vi "Gel Tugging Displacement Mode v.16.00.vi"() -> ()   [LabVIEW 2015]
doc: "This example demonstrates how to continuously acquire voltage measurements from a DAQmx device using hardware timed, single point reads using a timed loop structure. The timed loop is controlled by the sample clock of the DAQ device. The device will read data on each tick of the sample clock. If an additional sample clock tick occurs before the current data point is read from the device or if the timed loop does not receive any sample clock ticks, a dialog will indicate that this has happened. \n\nHardware Timed Single Point acquisition works best when using a deterministic operating system (such as LabVIEW Real-Time). Because of the less deterministic nature of general purpose operating systems (such as Microsoft Windows), the software loop will not always take the exact same amount of time to execute, and this may lead to the occasional missed sample clock. \n\nFor instructions on how to connect your signals to the DAQ device, refer to your device documentation."
uses:
  <vilib>/Platform/TimedLoop/XDataNode/timing_clust.ctl
  <vilib>/Platform/TimedLoop/XDataNode/nitl_modes.ctl
  <vilib>/Platform/TimedLoop/XDataNode/wakeup.ctl
  <vilib>/DAQmx/read.llb/DAQmx Read (Analog 1D DBL NChan 1Samp).vi
  <vilib>/DAQmx/write.llb/DAQmx Write (Analog DBL 1Chan 1Samp).vi
  <vilib>/DAQmx/read.llb/DAQmx Read (Analog 2D DBL NChan NSamp).vi
  <vilib>/Analysis/baseanly.llb/Mean (DBL).vi
  <vilib>/DAQmx/create/channels.llb/DAQmx Create Channel (AI-Voltage-Basic).vi
  <vilib>/DAQmx/create/channels.llb/DAQmx Create Channel (AO-Voltage-Basic).vi
  <vilib>/DAQmx/configure/timing.llb/DAQmx Timing (Sample Clock).vi
  <vilib>/DAQmx/create/timing.llb/DAQmx Create Timing Source (Control Loop From Task).vi
  <vilib>/DAQmx/miscellaneous.llb/DAQmx Fill In Error Info.vi
  <vilib>/addons/control/pid/pid.llb/PID (DBL).vi
  <vilib>/platform/TimedLoop/XDataNode/XDataNode.xnode
  <vilib>/Analysis/NI_AALBase.lvlib
  <vilib>/addons/control/pid/NI_PID_pid.lvlib
  <vilib>/Platform/TimedLoop/XDataNode/XDNodeRunTimeDep.lvlib
  <vilib>/ptbypt/NI_PtbyPt.lvlib
panel:
  out "Calibrating Sensor":bool
  out "Waveform Graph":dbl[](graph)
  in  "2. Force Clamp?":bool
  in  "Measure Flux Sensor Zero?":bool=TRUE
  in  "4. Aggressiveness:":i32(listbox)
  out "of":i32
  in  "3. PID Parameters:":i32(listbox)
  out "Measured Magnetic Sensor 1 Zero, Mean (V)":dbl format="%_7g"
  out "Round:":i32
  out "Ready?":bool
  out "Sensor Sensitivity \n(V/Gs)":dbl
  in  "1. Sensor:":i32(listbox)
  out "Ready?":bool
  in  "2. Needle:":i32(listbox)
  in  "Proceed with Selection":bool
  out "Real-Time Flux Control Currently Running?":bool
  out "DeGaussing?":bool
  in  "Start DeGaussing":bool
  in  "Start Null Flux Adjustment":bool
  in  "1. Number of rounds":i32=2
  in  "3. Keep Null Flux Running \n       Until Next Step?":bool=TRUE
  in  "4. Stop Program":bool
  # "For Gel Tugging Experiments v16.00 (Force Clamp/Controlled Displacement Mode)"
  # "WARNING: This program crashes the first 2 or 3 times it runs after the target has been shut down. \nWARNING: Do NOT run the power supply unattended with the needle attached. Always look at the amount of current periodically."
  # "Step 0-1: Place the needle at Z ~ 5000 micron in the field of view. Inclincation Angle= 45º for HyMu80#1 Needle"
  # "Step 0-2: DeGauss Needle:"
  # "(Hit \"Enter\" \nor Toggle)"
  # "Step 0-3: Measure the Value of Flux Sensor \"Zero\"?"
  # "Yes"
  # "No"
  # "Step 1: Choose Sensor & \nNeedle/PID Parameters\nfor This Experiment:"
  # "Step 2: Adjust Flux: \n(in Real-Time)"
  # "OFF"
  # "ON"
  # "Yes"
  # "No"
  # "Make sure upper side of Rocker\n is pressed down before Program Starts"
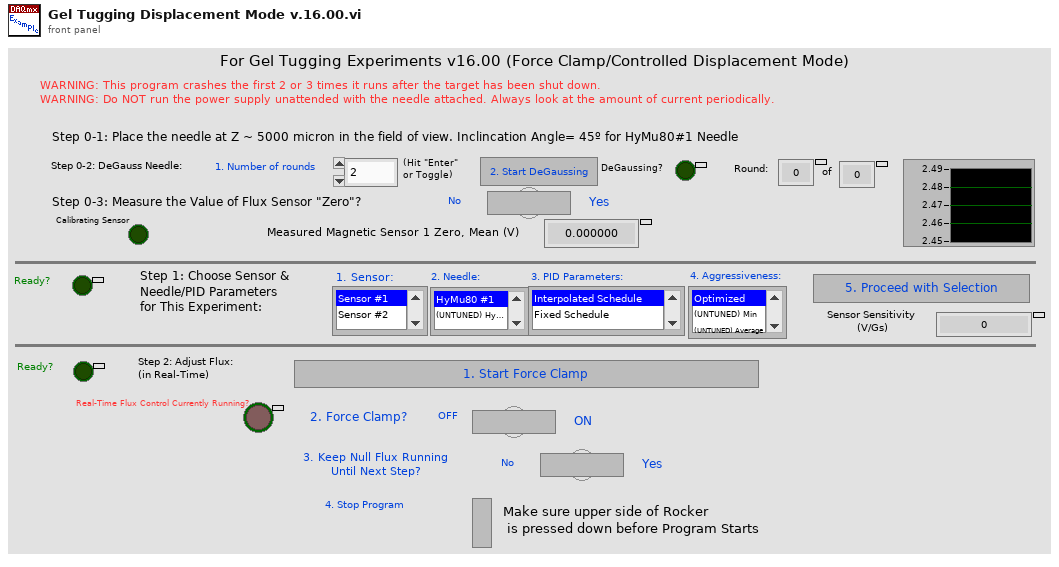
[diagram p1: front panel]
types:
  T1 = cluster{"PID gains":cluster{"proportional gain (Kc)":dbl, "integral time (Ti, min)":dbl, "derivative time (Td, min)":dbl}, "max value":dbl}[]
  T2 = typedef "XDNodeRunTimeDep.lvlib/timing_clust.ctl" = cluster{"Expected End [f-1]":u64, "Actual End [f-1]":u64, "Finished Late? [f-1]":bool, "Expected End [i-1]":u64, "Actual End [i-1]":u64, "Finished Late? [i-1]":bool, "Expected Start [i]":u64, "Actual Start [i]":u64, "Expected Start [f]":u64, "Actual Start [f]":u64, "Source Name":string, "Structure Name":string, "Period":i64, "Deadline":i64, "Offset":i64, "Start":i64, "Priority":i32, "Timeout":i32, "Mode":T3, "Wakeup Reason":T4, "Error":errorcluster, "Source Type":string, "Secondary Source Type":string, "Global End Time":u64, "Global Start Time":u64, "Frame Duration":u64, "Iteration Duration":u64, "Assigned CPU":i32, "I/O Scan Engine Mode":u32}
  T3 = typedef "XDNodeRunTimeDep.lvlib/nitl_modes.ctl" = enum32{"No Change", "Process missed periods, maintain original phase", "Discard missed periods, maintain original phase", "Process missed periods, ignore original phase", "Discard missed periods, ignore original phase"}
  T4 = typedef "XDNodeRunTimeDep.lvlib/wakeup.ctl" = enum32{"Normal", "Aborted", "Asynchronous wakeup", "Timing source error", "Timed loop error", "Timeout"}
  T5 = cluster{"proportional gain (Kc)":dbl, "integral time (Ti, min)":dbl, "derivative time (Td, min)":dbl}
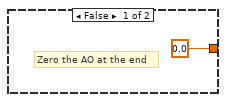
[diagram p2: hidden frame]
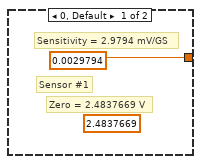
[diagram p4: hidden frame]
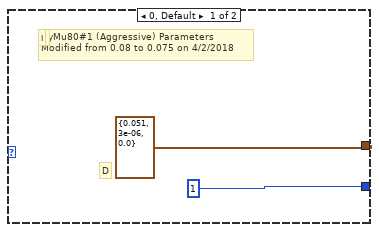
[diagram p5: hidden frame]
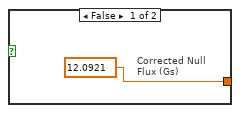
[diagram p6: hidden frame]
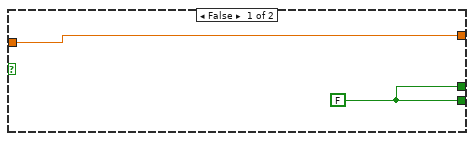
[diagram p7: hidden frame]
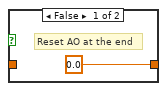
[diagram p8: hidden frame]
diagram:
  (unwired) T1 [{"PID gains"={"proportional gain (Kc)"=0.07, "integral time (Ti, min)"=3.5e-06, "derivative time (Td, min)"=0.0}, "max value"=0.0}, {"PID gains"={"proportional gain (Kc)"=0.07, "integral time (Ti, min)"=3.5e-06, "derivative time (Td, min)"=0.0}, "max value"=143.0}, {"PID gains"={"proportional gain (Kc)"=0.078, "integral time (Ti, min)"=3.5e-06, "derivative time (Td, min)"=0.0}, "max value"=148.0}, {"PID gains"={"proportional gain (Kc)"=0.078, "integral time (Ti, min)"=3.5e-06, "derivative time (Td, min)"=0.0}, "max value"=150.0}, {"PID gains"={"proportional gain (Kc)"=0.078, "integral time (Ti, min)"=3.5e-06, "derivative time (Td, min)"=0.0}, "max value"=155.0}, {"PID gains"={"proportional gain (Kc)"=0.078, "integral time (Ti, min)"=3.5e-06, "derivative time (Td, min)"=0.0}, "max value"=160.0}, {"PID gains"={"proportional gain (Kc)"=0.078, "integral time (Ti, min)"=3.5e-06, "derivative time (Td, min)"=0.0}, "max value"=165.0}, {"PID gains"={"proportional gain (Kc)"=0.078, "integral time (Ti, min)"=3.5e-06, "derivative time (Td, min)"=0.0}, "max value"=170.0}, {"PID gains"={"proportional gain (Kc)"=0.081, "integral time (Ti, min)"=3.5e-06, "derivative time (Td, min)"=0.0}, "max value"=175.0}, {"PID gains"={"proportional gain (Kc)"=0.081, "integral time (Ti, min)"=3.5e-06, "derivative time (Td, min)"=0.0}, "max value"=180.0}, {"PID gains"={"proportional gain (Kc)"=0.085, "integral time (Ti, min)"=3.5e-06, "derivative time (Td, min)"=0.0}, "max value"=185.0}, {"PID gains"={"proportional gain (Kc)"=0.086, "integral time (Ti, min)"=3.5e-06, "derivative time (Td, min)"=0.0}, "max value"=190.0}, {"PID gains"={"proportional gain (Kc)"=0.086, "integral time (Ti, min)"=0.01, "derivative time (Td, min)"=0.0}, "max value"=195.0}, {"PID gains"={"proportional gain (Kc)"=0.086, "integral time (Ti, min)"=0.01, "derivative time (Td, min)"=0.0}, "max value"=220.0}]  # OFF PID gain schedule HyMu80#1 Needle OPTIMIZED
  (unwired) T1 [{"PID gains"={"proportional gain (Kc)"=0.065, "integral time (Ti, min)"=3.5e-06, "derivative time (Td, min)"=0.0}, "max value"=0.0}, {"PID gains"={"proportional gain (Kc)"=0.065, "integral time (Ti, min)"=3.5e-06, "derivative time (Td, min)"=0.0}, "max value"=143.0}, {"PID gains"={"proportional gain (Kc)"=0.083, "integral time (Ti, min)"=3.5e-06, "derivative time (Td, min)"=0.0}, "max value"=148.0}, {"PID gains"={"proportional gain (Kc)"=0.084, "integral time (Ti, min)"=3.5e-06, "derivative time (Td, min)"=0.0}, "max value"=150.0}, {"PID gains"={"proportional gain (Kc)"=0.0875, "integral time (Ti, min)"=3.5e-06, "derivative time (Td, min)"=0.0}, "max value"=155.0}, {"PID gains"={"proportional gain (Kc)"=0.123, "integral time (Ti, min)"=3.5e-06, "derivative time (Td, min)"=0.0}, "max value"=160.0}, {"PID gains"={"proportional gain (Kc)"=0.187, "integral time (Ti, min)"=3.5e-06, "derivative time (Td, min)"=0.0}, "max value"=165.0}, {"PID gains"={"proportional gain (Kc)"=0.315, "integral time (Ti, min)"=3.5e-06, "derivative time (Td, min)"=0.0}, "max value"=170.0}, {"PID gains"={"proportional gain (Kc)"=0.46, "integral time (Ti, min)"=3.5e-06, "derivative time (Td, min)"=0.0}, "max value"=175.0}, {"PID gains"={"proportional gain (Kc)"=0.59, "integral time (Ti, min)"=3.5e-06, "derivative time (Td, min)"=0.0}, "max value"=180.0}, {"PID gains"={"proportional gain (Kc)"=0.8875, "integral time (Ti, min)"=3.5e-06, "derivative time (Td, min)"=0.0}, "max value"=185.0}, {"PID gains"={"proportional gain (Kc)"=1.04, "integral time (Ti, min)"=3.5e-06, "derivative time (Td, min)"=0.0}, "max value"=190.0}, {"PID gains"={"proportional gain (Kc)"=1.04, "integral time (Ti, min)"=0.01, "derivative time (Td, min)"=0.0}, "max value"=195.0}, {"PID gains"={"proportional gain (Kc)"=1.04, "integral time (Ti, min)"=0.01, "derivative time (Td, min)"=0.0}, "max value"=220.0}]  # ON PID gain schedule HyMu80#1 Needle OPTIMIZED
  (unwired) T1 [{"PID gains"={"proportional gain (Kc)"=0.07, "integral time (Ti, min)"=3.5e-06, "derivative time (Td, min)"=0.0}, "max value"=0.0}, {"PID gains"={"proportional gain (Kc)"=0.07, "integral time (Ti, min)"=3.5e-06, "derivative time (Td, min)"=0.0}, "max value"=116.0}, {"PID gains"={"proportional gain (Kc)"=0.078, "integral time (Ti, min)"=3.5e-06, "derivative time (Td, min)"=0.0}, "max value"=117.0}, {"PID gains"={"proportional gain (Kc)"=0.08, "integral time (Ti, min)"=3.5e-06, "derivative time (Td, min)"=0.0}, "max value"=120.0}, {"PID gains"={"proportional gain (Kc)"=0.08, "integral time (Ti, min)"=3.5e-06, "derivative time (Td, min)"=0.0}, "max value"=122.0}, {"PID gains"={"proportional gain (Kc)"=0.08, "integral time (Ti, min)"=3.5e-06, "derivative time (Td, min)"=0.0}, "max value"=125.0}, {"PID gains"={"proportional gain (Kc)"=0.08, "integral time (Ti, min)"=3.5e-06, "derivative time (Td, min)"=0.0}, "max value"=130.0}, {"PID gains"={"proportional gain (Kc)"=0.08, "integral time (Ti, min)"=3.5e-06, "derivative time (Td, min)"=0.0}, "max value"=135.0}, {"PID gains"={"proportional gain (Kc)"=0.08, "integral time (Ti, min)"=3.5e-06, "derivative time (Td, min)"=0.0}, "max value"=140.0}, {"PID gains"={"proportional gain (Kc)"=0.086, "integral time (Ti, min)"=3.5e-06, "derivative time (Td, min)"=0.0}, "max value"=145.0}, {"PID gains"={"proportional gain (Kc)"=0.096, "integral time (Ti, min)"=3.5e-06, "derivative time (Td, min)"=0.0}, "max value"=150.0}, {"PID gains"={"proportional gain (Kc)"=0.096, "integral time (Ti, min)"=3.5e-06, "derivative time (Td, min)"=0.0}, "max value"=200.0}]  # OFF PID gain schedule HyMu80#1 Needle OPTIMIZED
  (unwired) T1 [{"PID gains"={"proportional gain (Kc)"=0.07, "integral time (Ti, min)"=3.5e-06, "derivative time (Td, min)"=0.0}, "max value"=0.0}, {"PID gains"={"proportional gain (Kc)"=0.07, "integral time (Ti, min)"=3.5e-06, "derivative time (Td, min)"=0.0}, "max value"=116.0}, {"PID gains"={"proportional gain (Kc)"=0.08, "integral time (Ti, min)"=3.5e-06, "derivative time (Td, min)"=0.0}, "max value"=117.0}, {"PID gains"={"proportional gain (Kc)"=0.085, "integral time (Ti, min)"=3.5e-06, "derivative time (Td, min)"=0.0}, "max value"=120.0}, {"PID gains"={"proportional gain (Kc)"=0.115, "integral time (Ti, min)"=3.5e-06, "derivative time (Td, min)"=0.0}, "max value"=122.0}, {"PID gains"={"proportional gain (Kc)"=0.18, "integral time (Ti, min)"=3.5e-06, "derivative time (Td, min)"=0.0}, "max value"=125.0}, {"PID gains"={"proportional gain (Kc)"=0.31, "integral time (Ti, min)"=3.5e-06, "derivative time (Td, min)"=0.0}, "max value"=130.0}, {"PID gains"={"proportional gain (Kc)"=0.55, "integral time (Ti, min)"=3.5e-06, "derivative time (Td, min)"=0.0}, "max value"=135.0}, {"PID gains"={"proportional gain (Kc)"=0.95, "integral time (Ti, min)"=3.5e-06, "derivative time (Td, min)"=0.0}, "max value"=140.0}, {"PID gains"={"proportional gain (Kc)"=1.2, "integral time (Ti, min)"=3.5e-06, "derivative time (Td, min)"=0.0}, "max value"=145.0}, {"PID gains"={"proportional gain (Kc)"=1.3, "integral time (Ti, min)"=3.5e-06, "derivative time (Td, min)"=0.0}, "max value"=150.0}, {"PID gains"={"proportional gain (Kc)"=1.3, "integral time (Ti, min)"=3.5e-06, "derivative time (Td, min)"=0.0}, "max value"=200.0}]  # ON PID gain schedule HyMu80#1 Needle OPTIMIZED
  # "Re-optimized on 3/21/2018 for HyMu80#1 after shielding the sensor. The cutoff values were shifted down by ~23-27 Gs\nPreviously Optimized on 3/17/2018 for HyMu80#1 Optimized. The rest will need to be updated later\nAdded 139 Gs to keep fixed values in between 0 and 140 Gs.   Flux at 150 Gs has a response time of ~80 ms. \nAny higher PID gains will result in spike"
  # "Unshielded Previously"
  # "TOTALLY SHIELDED PARAMETERS"
  # "Note: Some quirks when running the program are: (as of 2/7/2018):\n1. First time you run it for the day, it will ask if you want to use the newer version instead of the old one already on the Remote Desktop computer\n2. Also, at the end of the first run, it will not stop. You will have to abort it. Some of the data points will be lost near the end. You might have to repeat that run.\n3. Do run the Data Reduction file or any other VIs in the DeGaussing stage. Otherwise, the program will crash."
  # "AI"
  # "AO"
  # "v16.00 modified from v15.10 by #Waddah Moghram on 1/12/2018:\n1. This is to be used with Force Clamp Mode Experiments. Flux values are -172 Gs and the Null Flux after magnetization in that order\n\nv15.10 modified from v15.00 by  #Waddah #Moghram on 11/5/2018 and therefore.\nTo be used with Data Logger v15.00 & Reduction v15.00: \n1. Modified it so that it can select PID gains from inside the loop\n2. Modified some PID gains at 170 Gs and higher.\n3.  Fixed the problem with the Post-wave zero Ramp 11/28/2019. WIM\n\nv 15.00 Modified from v12.00 by #Waddah #Moghram on 10/10/2018 and thereafter. To be used with Data Logger v1500 & Reduction v15.00: \n1. Replaced the Mini-DeGauss Routine with a Force Ramp (Linear vs. Steps?) since a step force function will be difficult to image-track. \n((Please refer to Linear and Step Ramps v1.00.vi for both linear and step ramps).\n*** Amount of step jump is assumed to be from ON-to-OFF and OFF-to-ON. That information is known\n2. Some of the parameters that will be used for the force ramp:\n*** Time interval: Assume that ON-to-OFF and OFF-to-ON ramps will have the same time frames.\n*** If discrete step are chosen. Choose the number of steps that it will take.\n\nv 11.00 Modified from v10.00 by #Waddah #Moghram on 4/26/2018 and thereafter. To be used with Data Logger v11.00 & Reduction v11.00: \n1. Resolve the issue of Digital Trigger automatically being released due to ground loop. Most likely due to construction that is happening around.\n* The Network digital trigger is released from the Master DAQ in the Data Logger, where it will be passed into here as a real-time global variable.\n2. For some reason, the first two runs usually crash, and the program still crashes a lot. I need to find a work around this one. \n\nv 10.00 Modified from v9.60 and v9.40 by #Waddah #Moghram on 4/4/2018 and thereafter: To be used with Data Logger v10.00 & Reduction v10.00\n1. Increased DeGauss Cycle to 2,000 milliseconds from 500 ms.\n2. Corrected the Dialog Boxes\n3. Added a switch for the Corrective Null Flux on the front panel, display it and send it to the Data Logger\n4. Corrected Mini-DeGauss Sampling Glitch where it was wired to the sampling rate directly instead of the one adjusted by the period 4/4/2018\n5. Based on a sigmoidal curve fit 4/18/2018.\nThe Equation is Y = Vmax * X^h /(K_prime + X^h), where Vmax = 10.7369, h = 1.91107, and Kprime = 3499.9. (and K_half = 71.5294))\n\n\nv 9.60 Modified from v9.50 by #Waddah #Moghram on 4/1/2018: \n1. It will correct for the Null Flux shift based on the Sigmoidal Fit that was collected from bead in front of the needle data,\nbased on a sigmoidal curve fit 4/2/2018. Experiments conducted 3/29/2018-4/2/2018. \nThe Equation is Y = Vmax * X^h /(K_prime + X^h), where Vmax = 11.4533, h = 1.69622, and Kprime = 1256.11)\n2. New Global Variable \"FluxObservedZeroGsCorrected\" to be inserted into the Data Logger v9.60\n\nv 9.50 Modified from v9.40 by #Waddah #Moghram on 3/29/2018:\n1. Used AI7 to hook up the 2nd Magnetic Sensor that will be placed in front of the sensor.\n2. Zero of 2nd Sensor is measured in the first step as well. The sensitivity is embedded in the data logger as well. \n3. Accompanies by v9.50 Data Logger.\n4. (GO BACK TO OLDER VERSION and add more details about modifications)\nFixed datapoints lost in the end due to the determinstic loop ending before the other loop. \n\nv 9.40 Modified from v9.20 by #Waddah #Moghram on 3/19/2018\n1. Removed Offset and kept amplitude +/- 10V for MiniDeGauss waveforms from inside the deterrministic loop.\n2. Shuffled the Suggested PID Loop parameters until before the \"Proceed button to allow the user to take a look at them. \n3. 3/22/2018. Reverted back to unshielded magnetic sensor, but with wire propped away from sensor.\nAlso, TI-SH-U is used and the needle is placed at Z~4600 microns for PID tuning with an inclination angle of 20 degrees\n(#OLD: 3. Re-optimized on 3/20/2018 for HyMu80#1 after shielding the sensor. The values were shifted down by 23 Gs   3/20/2018 )\n(#OLD: 4. Relocated PID Gains Selected on the front panel for more clarity 3/21/2018.)\n\nv 9.20 Modified from v9.05 and v9.10 by #Waddah #Moghram on 3/12/2018 and thereafter:\n1. It is back to OFF/ON Sequences, except first OFF segment and pre-waves have no DeGauss. It turns out to be an easy fix. \n2. Modified mini-DeGauss time \n3. Tied variables to make the wave sample properly. See notes for calculations.\n4. Turn OFF \"Null Flux Running Middle\" when control sequence starts. 3/17/2018 WIM \n5. Modified PID Parameters for #Interpolated #Optimized #HyMu80#1. Other parameters will need to be modified later on. \n6. Updated front panel to indicate inclination Angle, and Z-level for both Sensor Zero Measurement and Control Sequence.   3/18/2018\n****It turns out the PID parameters are sensitive to both z-level and inclination angle (which affect the Sensor Zero Measurement).*****\n***NOTE: First run usually does not end by itself. You will have to abort it. It will result in the loss of the last few hundred data points, but that is not too critical. Otherwise, run once, then run again. It should run smoothly every time afterwards. This is one of the quirks of working with LabVIEW. 3/18/2018\n\nv 9.05 Modified from v9.00 by #Waddah #Moghram on 3/12/2018:\n1. Modified Magnitude of Mini-DeGauss cycle from ** Maximum of (AO of Null Flux (AO_nf) or AO of ON (AO_on)) ** to **AO_nf + AO_on**\n2. The mini DeGauss oscillates about AO_nf instead of 0\n\nv 9.00 Modified from v8.40 by #Waddah #Moghram on 3/7/2018 and thereafter:\n1. It will include mini-DeGauss Cycles in the beginning of the OFF segments before PID control kicks back in. This is in an effort to minimize Magnetic Sensor hysteresis at Null Flux Observed\n(Sinusoidally Decaying Waveform Embedded in Control Sequence v1.0.vi is used for initially testing of mini-DeGauss waveforms).\n** So far, the selected waveform is about ~ 15 cycles that exponentially decay under 30 milliseconds. Used a Cosine waveform instead of sine (Sin with 90 degree phase shift).\n** Middle point is AO = 0, Magnitude between max and middle point is AO_last**    (3/12/2018)\n2. Sequence is created externally to minimize Loop calculation time. The AO Mini-DeGauss will only to be multiplied by the amplitude of the last AO out. \n3. Switched #AI6 to #AI3. Some errors with AI6 signal on the DAQ on 3/8/2018\n4. Fixed the glitch where the PID loop overreacted when the PID starts again and the Setpoint point is close to the Process variable. (Kudos to #Dr. #Selby for catching it!). on 3/8/2018\n5. Replaced \"Zero Flux\" with \"Null Flux\" for labels to avoid confusion since it is not really zero\n\nv 8.40 Modified from v8.30 by #Waddah #Moghram on 3/1/2018, and thereafter: \n1. Added a toggle to allow the re-calibration of magnetic sensor Zero or not\n2. Global Variables for DeGauss Cycles Total & Round\n3. Modified Tabbing order on 3/4/2018\n4. Fixed AO 0 initialized before PID loop to keep the value saved from \"keep Null Flux Running\" step on 3/5/2018. It was creating a blip in PID response. However, that does not seem to resolve the problem.\n\nv 8.30 Modified from v8.20 by #Waddah #Moghram on 2/22/2018:\n1. Using the measured magnetic sensor zero to create the control sequence after DeGaussing instead of the one recorded a while back inside a shielded data.\nThis is because it will change a lot over time with thermal drift and so forth. \n2. Reset the value of the sensor zero every time even no deGaussing was done.\n\nv 8.20 Modified from v8.10 by #Waddah #Moghram on 2/2/2018: \n1. This will allow the user to tweak the PID Parameters one more time before the actual experiment. This was found because it turns out that PID parameters can shift with time especially for values in the non-linear range.\n\nv. 8.10 Modified from v8.00 by #Waddah #Moghram on 1/10/2018 and thereafter:\n1. Scrapped fitted PID gains and used interpolated schedules in addition to schedules\n2. Updated PID Values for Gains and so forth.\n\nv 8.00 Modified from v7.40 by #Waddah #Moghram on 1/1/2018 and thereafter:\n1. Used the PID Gains from PID Tuning experiments \n2. Removed Normal vs. Aggressive and now will only use one set of parameters such that only one set of parameters are used\n3. Created a choice of Scheduled vs. Fitted Parameters. 1/8/2018.\n4. Fixed glitch that passed old values of waveform parameters to the global variable 1/8/2018. \n\nv 7.40 Modified from v 7.30 by #Waddah #Moghram on 12/22/2017 to including the following:\n1. Shifting the flux check and current reset only if DeGuassing Cycle required is not equal to zero. Otherwise, skip it, and keep the current running. I did this in case I need more than one run without removing the needle from the sample\n2. corrected total number of data points to allow for more than 2 seconds 1/4/2018 by #WIM\n\nv 7.30 Modified from v 7.20 by #Waddah #Moghram on 12/21/2017 to including the following:\n1. Removed Magnetic Flux Sensor Zero Calibration step, and embedded that value in the sensor section. The idea for doing that is that I want the flux values stated to be absolute. Thermal drift of sensor should not matter since PID should still work regardless of where the zero lies. Moreover, if I am accounting for the Null Flux observed, it should not matter what the absolute flux zero is.\n2. However, I kept the AO reset and used the AI2 to keep it running and also measured sensor values for 2 seconds to make sure that my values are controlled properly.\n3. Steps were re-numbered\n\nv 7.20 Modified from v7.10 by #Waddah #Moghram on 12/18/2017 to include the following:\n1. Custom-Length Waveforms. Data Reduction & Logger will be changed accordingly.\n2. Added Normal (~40 ms response time) vs. Aggressive (~22 ms response time) PID Parameters on 12/20/2017\n\nV 7.10 Modified from v7.00 by #Waddah #Moghram on 12/18/2017 to include the following:\n1. Switch order of DeGaussing & Calibrating Zero of Sensor. First Ensure that there is no residual magnetic. And secondly, reset AO just in case!\n\nv 7.00 Modified from v6.00 by #Waddah #Moghram on 12/18/2017 to include the following:\n1. Calibrated Null Flux at the beginning of the experiment without shielding to account for thermal drifts:\n*** Imported from \"01 Magnetic Sensor Zero Calibration v2.0 - Target.vi\"\n2. Included Second per Cycle\n3. Cleanup interface & Changed Step Numbers.\n\nv 6.00 Modified from v5.22 by #Waddah #Moghram on 12/5/2017 to include the following: \n1. Newer Magnetic Sensor Sensitivities: Sensor 1 is 2.9794 mV/GS and Sensor 2 is 3.0418 mV/GS\n2. Newer Magnetic Sensor Zeroes when unshielded: Sensor 1 is 2.4837669 V and Sensor 2 is 2.4928421 V\nThis program will also be used also to tune the PID in addition Magnetic Needle Choices\nOn 12/13/2017, I overhauled the interface to streamline the proceess and fixed a few glitches that allowed the program to \nchose parameters before clicking on the digital trigger\n\nv 5.22 Modified from v.5.20 by #Waddah #Moghram on 9/25/2017 to include the following:\n1. Remove prompt to calibrate the magnetic sensor and run Null Flux program\n2. Embedded the calibrated Null Flux value into the program, now that the sensor is fixed to the HyMu80 needle #1\n\n\nv5.00 modified from v.3.70 and v.4.10 by #Waddah #Moghram. It should integrate variables from both VIs.\nOther modification include:\n1. User-Defined Pre-experiment Null Flux Period\n2. User-Defined Post-experiment Null Flux Period\nModified on 8/14&15/2017 to streamline the VI even more. Ran into some Ground Loop Issues in the meantime. See Lab Notes for details.\n\nv4.10 Modified on 8/8/2017 to:\n* account for AI5 only for flux sensor values being fed to PID control.\nNotice the PID control scheme process variable is different in that it is not subtracted from the setpoint as in v.3.70 in the first PID Loop\n*modified PID parameters to the optimized ones found (subject to verification)."
  n1 = flat-sequence {
    tunnel: [w245] -> w16
    tunnel: [w244] -> w15
    tunnel: [w243] -> w11
    tunnel: [w242] -> w4
    tunnel: [w257] -> w19
    tunnel: w16 -> [w255]
    tunnel: w15 -> [w254]
    tunnel: w11 -> [w253]
    tunnel: [w253] -> w10
    tunnel: [w252] -> w5
    tunnel: w4 -> [w252]
    tunnel: [w267] -> w20
    tunnel: w19 -> [w267]
    tunnel: w10 -> [w266]
    tunnel: [w266] -> w9
    tunnel: [w265] -> w6
    tunnel: w5 -> [w265]
    tunnel: w20 -> [w273]
    tunnel: [w272] -> w17
    tunnel: [w271] -> w13
    tunnel: w9 -> [w271]
    tunnel: [w270] -> w7
    tunnel: w6 -> [w270]
    tunnel: [w284] -> w26
    tunnel: [w283] -> w25
    tunnel: [w282] -> w24
    tunnel: [w281] -> w18
    tunnel: w17 -> [w281]
    tunnel: w13 -> [w280]
    tunnel: [w280] -> w12
    tunnel: [w278] -> w8
    tunnel: w7 -> [w279]
    tunnel: [w279] -> w3
    tunnel: w26 -> [w326]
    tunnel: w25 -> [w325]
    tunnel: w24 -> [w324]
    tunnel: [w323] -> w23
    tunnel: [w322] -> w22
    tunnel: [w321] -> w21
    tunnel: w18 -> [w312]
    tunnel: [w310] -> w14
    tunnel: w12 -> [w310]
    tunnel: w8 -> [w309]
    tunnel: w3 -> [w308]
    tunnel: [w308] -> w2
    tunnel: [w307] -> w1
    tunnel: w23 -> [w401]
    tunnel: w22 -> [w400]
    tunnel: w21 -> [w399]
    tunnel: w14 -> [_]
    tunnel: w2 -> [_]
    tunnel: w1 -> [_]
    frame #0 {
      # "Removed the thermocouple  * AI2 is connected to Thermocouple cable."
      # "Switched Ai6 to AI3 on 3/8/2018 \nSome issues with AI6 on DEV2"
      # "1. SPECIFY the number of DeGaussing Cycle. CLICK \"Start DeGaussing.\"\n2. SPECIFY the Sensor & Needle in use for this experiment."
      n2 = One Button Dialog(message="BEFORE YOU START: \n* VERIFY these DAQ-2/Slave cables are connected as the following:\n   * AI5 is connected to Magnetic Flux \"Sensor Output - RAW\" on the Magnetic sensor box.   \n   * AI3 is connected to \"Current Sensor (1A/V)\" on the Load Box.\n   * AI7 is connected to Camera \"Exposure Sensor.\"\n   * Digital Trigger from DAQ-3/Master Output \"PF0.0\" is connected to Digital Trigger Input \"PFI0.\"\n* VERIFY these DAQ-3/Master Cables are connected as the following:\n   * Digital Trigger is connected to \"PF0.0\" BOTH \"PFI0\" on the same board and to \"PFI0\" on DAQ2/Slave.\n  \n* TURN ON power supply for half an hour. TURN ON fan control for load box (if needed).\n           WARNING: Check load is connected at the back of the load box to the back of the  power supply.\n           WARNING: Check if magnetic coil is connected to the load box if the toggle is switched to \"COIL+1OHM RESISTOR\" on the Load Box.\n           WARNING: Do NOT Position Needle in solution/cells just yet.\n           WARNING: Do NOT Position Needle in solution/cells just yet.\nIf you have not done these steps. Stop the program, then run it when ready.\n===============================\nClick OK then follow the steps", button name ("OK")="OK!") -> ()  [unwired: 1 out]
    }
    frame #1 {
      (unwired) i8 0 ("Sensor Index Flux Core")
      w41 = tag "Dev2/ai4, Dev2/ai5, Dev2/ai7, Dev2/ai2, Dev2/ai3"  # AI2:Dummy,AI3: Current, AI4: Dummy,AI5:Flux, AI7: Camera  (VERY BAD @ 10k Zero. VERY GOOD otherwise)
      (unwired) tag "Dev2/ai4, Dev2/ai5, Dev2/ai7, Dev2/ai2, Dev2/ai3" ("AI2:Dummy,AI3: Current, AI4: Dummy,AI5:Flux, AI7: Camera \n(VERY BAD @ 10k Zero. VERY GOOD otherwise)")
      (unwired) tag "Dev2/ai5, Dev2/ai7, Dev2/ai3" ("AI2:Dummy,AI3: Current, AI4: Dummy,AI5:Flux, AI7: Camera \n(VERY BAD @ 10k Zero. VERY GOOD otherwise)")
      w31 = 0.0 ("DataRT Index")
      w37 = FALSE ("DeGuassing Needle")
      # "Added on 4/24/2018"
      # "RESET VARIABLES"
      n3 = shared-variable "NI-GenericDesktopPC-3A84958E\\Kopco PS Project Target Variables Library.lvlib\\Needle Selection Finished"(w37) -> ()  [unwired: 1 in, 1 out]
      n4 = shared-variable "NI-GenericDesktopPC-3A84958E\\Kopco PS Project Target Variables Library.lvlib\\Control Parameters Selected"(w37) -> ()  [unwired: 1 in, 1 out]
      n5 = shared-variable "NI-GenericDesktopPC-3A84958E\\Kopco PS Project Target Variables Library.lvlib\\DeGuassing Finished"(w37) -> ()  [unwired: 1 in, 1 out]
      n6 = shared-variable "NI-GenericDesktopPC-3A84958E\\Kopco PS Project Target Variables Library.lvlib\\DeGuassing Needle"(w37) -> ()  [unwired: 1 in, 1 out]
      n7 = shared-variable "NI-GenericDesktopPC-3A84958E\\Kopco PS Project Target Variables Library.lvlib\\Null Flux Selected"(w37) -> ()  [unwired: 1 in, 1 out]
      n8 = shared-variable ".\\Kopco PS Project Target Variables Library.lvlib\\Data Upload"(w37) -> ()  [unwired: 1 in, 1 out]
      n9 = shared-variable "NI-GenericDesktopPC-3A84958E\\Kopco PS Project Target Variables Library.lvlib\\Flux RT Control"(w37) -> ()  [unwired: 1 in, 1 out]
      n10 = shared-variable "NI-GenericDesktopPC-3A84958E\\Kopco PS Project Target Variables Library.lvlib\\Flux Control Sequence Running"(w37) -> ()  [unwired: 1 in, 1 out]
      n11 = shared-variable "NI-GenericDesktopPC-3A84958E\\Kopco PS Project Target Variables Library.lvlib\\Null Flux Running Middle"(w37) -> ()  [unwired: 1 in, 1 out]
      n12 = shared-variable "NI-GenericDesktopPC-3A84958E\\Kopco PS Project Target Variables Library.lvlib\\Null Flux Running End"(w37) -> ()  [unwired: 1 in, 1 out]
      n13 = shared-variable "NI-GenericDesktopPC-3A84958E\\Kopco PS Project Target Variables Library.lvlib\\Zero Flux Calibrated Found"(w37) -> ()  [unwired: 1 in, 1 out]
      n14 = shared-variable "NI-GenericDesktopPC-3A84958E\\Kopco PS Project Target Variables Library.lvlib\\PID Parameters Selected"(w37) -> ()  [unwired: 1 in, 1 out]
      n15 = shared-variable "NI-GenericDesktopPC-3A84958E\\Kopco PS Project Target Variables Library.lvlib\\Digital Trigger"(w37) -> ()  [unwired: 1 in, 1 out]
      n16 = shared-variable ".\\Kopco PS Project Target Variables Library.lvlib\\Data RT Flux"(w31) -> ()  [unwired: 1 in, 1 out]
      n17 = shared-variable ".\\Kopco PS Project Target Variables Library.lvlib\\Data RT Exposure"(w31) -> ()  [unwired: 1 in, 1 out]
      n18 = shared-variable ".\\Kopco PS Project Target Variables Library.lvlib\\Data RT Current"(w31) -> ()  [unwired: 1 in, 1 out]
      n19 = shared-variable ".\\Kopco PS Project Target Variables Library.lvlib\\Data RT Index"(i64 0 ("DataRT Index")) -> ()  [unwired: 1 in, 1 out]
      n20 = shared-variable ".\\Kopco PS Project Target Variables Library.lvlib\\Last Current AO"(0.0 ("Last Current AO")) -> ()  [unwired: 1 in, 1 out]
      n21 = shared-variable "NI-GenericDesktopPC-3A84958E\\Kopco PS Project Target Variables Library.lvlib\\Experiment Settings Entered"(w37) -> ()  [unwired: 1 in, 1 out]
      n22 = shared-variable "NI-GenericDesktopPC-3A84958E\\Kopco PS Project Target Variables Library.lvlib\\Ramp Total Interval (ms)"(i16 0 ("Ramp Total Interval (ms)")) -> ()  [unwired: 1 in, 1 out]
      n23 = shared-variable "NI-GenericDesktopPC-3A84958E\\Kopco PS Project Target Variables Library.lvlib\\Ramp Steps"(i16 0 ("Ramp Steps")) -> ()  [unwired: 1 in, 1 out]
      n24 = shared-variable "NI-GenericDesktopPC-3A84958E\\Kopco PS Project Target Variables Library.lvlib\\DeGauss Round Num"(i16 0 ("DeGauss Round Num")) -> ()  [unwired: 1 in, 1 out]
      n25 = shared-variable "NI-GenericDesktopPC-3A84958E\\Kopco PS Project Target Variables Library.lvlib\\DeGauss Total"(i16 0 ("DeGauss Total")) -> ()  [unwired: 1 in, 1 out]
      n26 = shared-variable "NI-GenericDesktopPC-3A84958E\\Kopco PS Project Target Variables Library.lvlib\\Cycles"(i16 0 ("Cycles")) -> ()  [unwired: 1 in, 1 out]
      n27 = shared-variable "NI-GenericDesktopPC-3A84958E\\Kopco PS Project Target Variables Library.lvlib\\Channels AI List"(w41) -> ()  [unwired: 1 in, 1 out]
      n28 = shared-variable "NI-GenericDesktopPC-3A84958E\\Kopco PS Project Target Variables Library.lvlib\\Sampling Rate"(30000.0 ("Sampling Rate")) -> ()  [unwired: 1 in, 1 out]
      n29 = shared-variable "NI-GenericDesktopPC-3A84958E\\Kopco PS Project Target Variables Library.lvlib\\Sensor Index Flux Core"(i8 1 ("Sensor Index Flux Core")) -> ()  [unwired: 1 in, 1 out]
      n30 = shared-variable "NI-GenericDesktopPC-3A84958E\\Kopco PS Project Target Variables Library.lvlib\\Sensor Index Camera"(i8 2 ("Sensor Index Flux Core")) -> ()  [unwired: 1 in, 1 out]
      n31 = shared-variable "NI-GenericDesktopPC-3A84958E\\Kopco PS Project Target Variables Library.lvlib\\Sensor Index Current"(i8 4 ("Sensor Index Flux Core")) -> ()  [unwired: 1 in, 1 out]
    }
    frame #2 {
      # "#STEP #0"
      n32 = while {
        tunnel: ["Start DeGaussing"] -> w43
        stop <- "Start DeGaussing" stop-if-true
      }
      n33 = shared-variable "NI-GenericDesktopPC-3A84958E\\Kopco PS Project Target Variables Library.lvlib\\DeGuassing Needle"(w43) -> ()  [unwired: 1 in, 1 out]
    }
    frame #3 {
      # "bound to \n\"DeGaussing Needle\"\nshared global variable"
      # "Bound to \n\"DeGauss Round Num\""
      # "Bound to \"DeGauss Total\""
      n34 = shared-variable "NI-GenericDesktopPC-3A84958E\\Kopco PS Project Target Variables Library.lvlib\\DeGauss Total"("1. Number of rounds") -> ()  [unwired: 1 in, 1 out]
      n35 = for {
        N: "1. Number of rounds" -> [_]
        i -> [w52]
        # "Wait half a second\nbetween repititions \nto allow the system \nto stabilize\n\nAdded by WIM on \n12/18/2017\n\nUpdated to 2 Seconds\nfrom 500 ms"
        # "First Index is 0"
        n36 = Add(x=1, y=w52) -> (x+y=w46:i32)
        n37 = shared-variable "NI-GenericDesktopPC-3A84958E\\Kopco PS Project Target Variables Library.lvlib\\DeGauss Round Num"(w46) -> ()  [unwired: 1 in, 1 out]
        n38 = Wait (ms)(milliseconds to wait=u32 2000) -> ()  [unwired: 1 out]
        n39 = flat-sequence {
          tunnel: [w65] -> w61
          tunnel: [w63] -> w60
          tunnel: w46 -> [w64]
          tunnel: [w64] -> w49
          tunnel: w61 -> [w87]
          tunnel: [w94] -> w59
          tunnel: [w86] -> w58
          tunnel: [w100] -> w57
          tunnel: w60 -> [w85]
          tunnel: [w85] -> w56
          tunnel: w49 -> [w84]
          tunnel: [w84] -> w48
          tunnel: w59 -> [w117]
          tunnel: w58 -> [w118]
          tunnel: w57 -> [w125]
          tunnel: [w124] -> w55
          tunnel: [w123] -> w54
          tunnel: [w122] -> w53
          tunnel: w56 -> [w115]
          tunnel: w48 -> [w113]
          tunnel: [w113] -> w47
          tunnel: w55 -> [w160]
          tunnel: w54 -> [w159]
          tunnel: w53 -> [w155]
          tunnel: w47 -> [_]
          frame #0 {
            w66 = 5  # Time in Seconds
            w65 = 6000  # Sampling Rate (Samples/Seconds)
            # "Step 0 DeGaussing"
            # "Hardware-Time control loop cannot keep up\nwith 50,000 Hz frequence."
            n40 = Multiply(x=w66, y=w65) -> (x*y=w67:i32)
            n41 = Decrement(x=w67) -> (x-1=w62:i32)
            n42 = for "A Single DeGuassing Waveform" {
              N: w62 -> [_]
              tunnel: w65 -> [w71]
              tunnel: [w68] -> w63 mode=indexing
              i -> [w70]
              (unwired) 0.3 ("y")
              w74 = 1.0  # A_0
              w77 = 1.0  # Lambda
              w81 = 0.0  # No phase
              w82 = 60.0  # Frequency, 60 Hz
              w83 = 10.0  # 4 amps = 10V
              # "Minimized 10 V to 5 V on 3/19/2018\nadd an offset of 0.3V for now"
              # "Lambda = ln(2)/(halflife time)^2"
              n43 = To Double Precision Float(number=w70) -> (double precision float=w72:dbl)
              n44 = Divide "dT"(x=w72, y=w71) -> (x/y=w69:dbl)
              n45 = Square(x=w69) -> (x^2=w75:dbl)
              n46 = Negate(x=w75) -> (-x=w76:dbl)
              n47 = call <vilib>:"Sine Wave PtByPt.vi"("time"=w69, "phase"=w81, "frequency"=w82, "amplitude"=w83) -> ("sine wave"=w80:dbl)
              n48 = Divide(x=w76, y=w77) -> (x/y=w78:dbl)
              n49 = Exponential(1:w78) -> (0:w79:dbl)
              n50 = Multiply(x=w79, y=w74) -> (x*y=w73:dbl)
              n51 = Multiply(x=w80, y=w73) -> (x*y=w68:dbl)
            }
          }
          frame #1 {
            w95 = -1 items=["default"=-1, "RSE"=10083, "NRSE"=10078, "Differential"=10106, "Pseudodifferential"=12529] ("Terminal Configuration")
            w101 = 12522 items=["Finite Samples"=10178, "Continuous Samples"=10123, "Hardware Timed Single Point"=12522]  # Sample Mode
            w108 = 10106 items=["default"=-1, "RSE"=10083, "NRSE"=10078, "Differential"=10106, "Pseudodifferential"=12529] ("Terminal Configuration")
            w111 = 12522 items=["Finite Samples"=10178, "Continuous Samples"=10123, "Hardware Timed Single Point"=12522]  # Sample Mode
            # "Step 0 DeGaussing"
            # "Power Supply Control"
            # "Magnetic Flux Sensor Signals\nOnly initiated to control \ndeterministic loop"
            n52 = call-poly <vilib>:"DAQmx Create Virtual Channel.vi"("maximum value"=5.0 ("Max Voltage"), "minimum value"=0.0 ("Min Voltage"), "input terminal configuration"=w108, "physical channels"="Dev2/ai5") -> ("task out"=w109:refnum<k21>, "error out"=w110:errorcluster)  [unwired: 10 in]
            n53 = call-poly <vilib>:"DAQmx Create Virtual Channel.vi"("maximum value"=10.0, "minimum value"=-10.0, "output terminal configuration"=w95, "physical channels"="Dev2/ao0") -> ("task out"=w105:refnum<k21>, "error out"=w104:errorcluster)  [unwired: 10 in]
            n54 = call-poly <vilib>:"DAQmx Timing.vi"("task/channels in"=w109, "sample mode"=w111, "rate"=w87, "error in"=w110) -> ("task out"=w98:refnum<k21>, "error out"=w93:errorcluster)  [unwired: 10 in]
            n55 = call "Get Terminal Name with Device Prefix.vi"("error in"=w93, "Local Terminal Name"="ai/SampleClock", "task/channels in"=w98) -> ("error out"=w92:errorcluster, "Terminal Name with Device Prefix"=w91:tag, "task out"=w94:refnum<k21>)  [unwired: 6 in]
            n56 = call-poly <vilib>:"DAQmx Timing.vi"("task/channels in"=w105, "sample mode"=w101, "rate"=w87, "source"=w91, "error in"=w104) -> ("task out"=w88:refnum<k21>, "error out"=w89:errorcluster)  [unwired: 9 in]
            n57 = call <vilib>:"DAQmx Start Task.vi"("task/channels in"=w88, "error in"=w89) -> ("task out"=w100:refnum<k21>, "error out"=w99:errorcluster)  [unwired: 12 in]
            n58 = Merge Errors(w92, w99) -> (w86:errorcluster)
          }
          frame #2 {
            # "Step 0 DeGaussing"
            n59 = call-poly <vilib>:"DAQmx Create Timing Source.vi"("task/channels in"=w117, "sleep time (us)"=1.0, "error in"=w118) -> ("task out"=w114:refnum<k21>, "timing source out"=w116:string, "error out"=w112:errorcluster)  [unwired: 10 in]
            n60 = node-c288(w116, w112) -> (w121:T2)  [unwired: 8 in]
            n61 = timed-loop "DeGuassing Control" {
              tunnel: w114 -> [w144]
              tunnel: [w137] -> w123
              tunnel: w125 -> [w127]
              tunnel: [w142] -> w122
              tunnel: w112 -> [w141]
              tunnel: [w140] -> w124
              timing: w121 -> [_]
              timing-out: [_] -> w120
              tunnel: w115 -> [w129]
              i -> [w133]
              stop <- w126 continue-if-true
              # "PS does not turn off unless two values are written."
              # "Offset by 1 to eliminate\nextra datapoint at end"
              n62 = node-c288() -> ()  [unwired: 1 in, 1 out]
              n63 = Array Size(array=w129) -> (size(s)=w134:i32)
              n64 = Index Array "Index Array"(array=w129, index=w133) -> (element=w130:dbl)
              n65 = call-poly <vilib>:"DAQmx Read.vi"("task/channels in"=w144, "error in"=w141) -> ("task out"=w137:refnum<k21>, "error out"=w143:errorcluster)  [unwired: 11 in, 1 out]
              n66 = Less?(x=w133, y=w134) -> (x < y?=w132:bool)
              n67 = Subtract(x=w134, y=2) -> (x-y=w136:i32)
              n68 = Less?(x=w133, y=w136) -> (x < y?=w131:bool)
              n69 = case shown="True" w131 {
                tunnel: [0.0 ("output") w147] -> w128
                tunnel: w130 -> [_ w147]
                frame False {
                  # "Zero the AO at the end"
                }
                frame True {
                }
              }
              n70 = call-poly <vilib>:"DAQmx Write.vi"("task/channels in"=w127, "data"=w128, "error in"=w143) -> ("task out"=w142:refnum<k21>, "error out"=w140:errorcluster)  [unwired: 10 in, 1 out]
              n71 = Unbundle By Name(w140) -> ("status"=w145:bool)  [unwired: 2 out]
              n72 = Not Or(1:FALSE ("Stop"), 2:w145) -> (0:w138:bool)
              n73 = And(x=w138, y=w132) -> (x .and. y?=w126:bool)
              n74 = shared-variable "NI-GenericDesktopPC-3A84958E\\Kopco PS Project Target Variables Library.lvlib\\DeGuassing Needle"(w126) -> ()  [unwired: 1 in, 1 out]
              n75 = node-c288() -> ()  [unwired: 1 in, 1 out]
            }
            n76 = node-c288(w120) -> ()  [unwired: 1 out]
          }
          frame #3 {
            n77 = call <vilib>:"DAQmx Stop Task.vi"("task/channels in"=w159, "error in"=w160) -> ("task out"=w162:refnum<k21>, "error out"=w161:errorcluster)  [unwired: 12 in]
            n78 = call <vilib>:"DAQmx Clear Task.vi"("task in"=w162, "error in"=w161) -> ("error out"=w156:errorcluster)  [unwired: 13 in]
            n79 = call <vilib>:"DAQmx Stop Task.vi"("task/channels in"=w155, "error in"=w156) -> ("task out"=w158:refnum<k21>, "error out"=w157:errorcluster)  [unwired: 12 in]
            n80 = call <vilib>:"DAQmx Clear Task.vi"("task in"=w158, "error in"=w157) -> ()  [unwired: 13 in, 1 out]
          }
        }
      }
    }
    frame #4 {
      # "Step 0 Reset the Magnetic Sensor"
      n81 = case shown="True" "Measure Flux Sensor Zero?" {
        frame False {
        }
        frame True {
          w171 = 12522 items=["Finite Samples"=10178, "Continuous Samples"=10123, "Hardware Timed Single Point"=12522] ("sample mode")
          w185 = 3.0  # Time (s)
          w184 = 10000  # Samples read  per loop
          w204 = -1 items=["default"=-1, "RSE"=10083, "NRSE"=10078, "Differential"=10106, "Pseudodifferential"=12529] ("Terminal Configuration")
          w201 = 12522 items=["Finite Samples"=10178, "Continuous Samples"=10123, "Hardware Timed Single Point"=12522]  # Sample Mode
          w193 = 10106 items=["Default"=-1, "RSE"=10083, "NRSE"=10078, "Differential"=10106, "Pseudodifferential"=12529]  # input terminal configuration
          w196 = 0
          # "Changed on 3/29/2018 to include Sensor 2 placed in front of the needle. Added Global Variable \"Flux Calibrated Zero 2\""
          # "Reset AO to 0. Sometimes it overshoot after DeGaussing\nAdded by #WIM on 12/18/2017"
          # "Power Supply Control"
          n82 = shared-variable "NI-GenericDesktopPC-3A84958E\\Kopco PS Project Target Variables Library.lvlib\\Channels AI List"() -> (w187:string)  [unwired: 1 in, 1 out]
          n83 = shared-variable "NI-GenericDesktopPC-3A84958E\\Kopco PS Project Target Variables Library.lvlib\\Sampling Rate"() -> (w166:dbl)  [unwired: 1 in, 1 out]
          n84 = call-poly <vilib>:"DAQmx Create Virtual Channel.vi"("maximum value"=5.0, "minimum value"=0.0, "input terminal configuration"=w193, "physical channels"=w187) -> ("task out"=w167:refnum<k21>, "error out"=w168:errorcluster)  [unwired: 10 in]
          n85 = call-poly <vilib>:"DAQmx Create Virtual Channel.vi"("maximum value"=10.0, "minimum value"=-10.0, "output terminal configuration"=w204, "physical channels"="Dev2/ao0") -> ("task out"=w198:refnum<k21>, "error out"=w199:errorcluster)  [unwired: 10 in]
          n86 = call-poly <vilib>:"DAQmx Timing.vi"("task/channels in"=w167, "sample mode"=w171, "rate"=w166, "error in"=w168) -> ("task out"=w170:refnum<k21>, "error out"=w169:errorcluster)  [unwired: 10 in]
          n87 = Multiply "Total Samples \nper Channel"(x=w166, y=w185) -> (x*y=w186:dbl)
          n88 = call "Get Terminal Name with Device Prefix.vi"("error in"=w169, "Local Terminal Name"="ai/SampleClock", "task/channels in"=w170) -> ("error out"=w181:errorcluster, "Terminal Name with Device Prefix"=w180:tag, "task out"=w176:refnum<k21>)  [unwired: 6 in]
          n89 = call-poly <vilib>:"DAQmx Timing.vi"("task/channels in"=w198, "sample mode"=w201, "rate"=w166, "source"=w180, "error in"=w199) -> ("task out"=w206:refnum<k21>, "error out"=w205:errorcluster)  [unwired: 9 in]
          n90 = call <vilib>:"DAQmx Start Task.vi"("task/channels in"=w206, "error in"=w205) -> ("task out"=w209:refnum<k21>, "error out"=w208:errorcluster)  [unwired: 12 in]
          n91 = Merge Errors(w181, w208) -> (w174:errorcluster)
          n92 = Subtract "Almost Total"(x=w186, y=w184) -> (x-y=w183:dbl)
          n93 = shared-variable "NI-GenericDesktopPC-3A84958E\\Kopco PS Project Target Variables Library.lvlib\\Sensor Index Flux Core"() -> (w165:i8)  [unwired: 1 in, 1 out]
          n94 = call-poly <vilib>:"DAQmx Create Timing Source.vi"("task/channels in"=w176, "sleep time (us)"=1.0, "error in"=w174) -> ("task out"=w177:refnum<k21>, "timing source out"=w172:string, "error out"=w175:errorcluster)  [unwired: 10 in]
          n95 = Initialize Array(w196, w196) -> (w189:i32[])
          n96 = node-c288(w172) -> (w179:T2)  [unwired: 3 in]
          n97 = timed-loop {
            tunnel: w177 -> [w230]
            tunnel: w175 -> [w225]
            tunnel: [w231] -> w213
            shift-right: [w232] -> _
            shift-left: 0 -> [w233]
            tunnel: [w229] -> w207
            shift-right: [w227] -> w164
            shift-left: w189 -> [w222]
            tunnel: [w222] -> _
            tunnel: w209 -> [w226]
            tunnel: [w221] -> w214
            tunnel: w184 -> [w219]
            tunnel: w183 -> [w218]
            timing: w179 -> [_]
            timing-out: [_] -> w178
            shift-right: [w217] -> _
            shift-left: _ -> [_]
            tunnel: w165 -> [w215]
            i -> [w217]
            stop <- w216 continue-if-true
            w234 = 10.0  # timeout
            # "Magnetic Sensor 2"
            # "Magnetic Sensor 1"
            n98 = node-c288() -> ()  [unwired: 1 in, 1 out]
            n99 = call-poly <vilib>:"DAQmx Write.vi"("task/channels in"=w226, "data"=0.0, "error in"=w225) -> ("task out"=w221:refnum<k21>, "error out"=w224:errorcluster)  [unwired: 10 in, 1 out]
            n100 = call-poly <vilib>:"DAQmx Read.vi"("task/channels in"=w230, "number of samples per channel"=w219, "timeout"=w234, "error in"=w224) -> ("task out"=w229:refnum<k21>, "data"=w220:dbl[][], "error out"=w231:errorcluster)  [unwired: 9 in]
            n101 = Add(x=w233, y=w219) -> (x+y=w232:i32)
            n102 = Unbundle By Name(w231) -> ()  [unwired: 1 out]
            n103 = Less Or Equal?(x=w232, y=w218) -> (x <= y?=w216:bool)
            n104 = Delete From Array(array=w220, index (row)=w215) -> (deleted portion=w228:dbl[])  [unwired: 2 in, 1 out]
            n105 = shared-variable "NI-GenericDesktopPC-3A84958E\\Kopco PS Project Target Variables Library.lvlib\\Sensor Zero Calibrating"(w216) -> ()  [unwired: 1 in, 1 out]
            n106 = Build Array (concatenate)(w222, w228) -> (w227:dbl[])
            n107 = node-c288() -> ()  [unwired: 1 in, 1 out]
          }
          "Waveform Graph" <- w164
          n108 = node-c288(w178) -> ()  [unwired: 1 out]
          n109 = call <vilib>:"Std Deviation and Variance.vi"("X"=w164) -> ("mean"=w190:dbl)  [unwired: 1 in, 2 out]
          n110 = call <vilib>:"DAQmx Stop Task.vi"("task/channels in"=w214, "error in"=w213) -> ("task out"=w210:refnum<k21>, "error out"=w211:errorcluster)  [unwired: 12 in]
          n111 = shared-variable "NI-GenericDesktopPC-3A84958E\\Kopco PS Project Target Variables Library.lvlib\\Zero Flux Calibrated Core"(w190) -> ()  [unwired: 1 in, 1 out]
          n112 = call <vilib>:"DAQmx Clear Task.vi"("task in"=w210, "error in"=w211) -> ("error out"=w212:errorcluster)  [unwired: 13 in]
          n113 = call <vilib>:"DAQmx Stop Task.vi"("task/channels in"=w207, "error in"=w212) -> ("task out"=w195:refnum<k21>, "error out"=w194:errorcluster)  [unwired: 12 in]
          n114 = call <vilib>:"DAQmx Clear Task.vi"("task in"=w195, "error in"=w194) -> ("error out"=w188:errorcluster)  [unwired: 13 in]
          n115 = call <vilib>:"General Error Handler.vi"("error in (no error)"=w188) -> ()  [unwired: 10 in, 5 out]
        }
      }
    }
    frame #5 {
      # "Bound to \"Flux Calibrated Zero 2\" \nglobal Variable"
      # "Bound to \"Flux Calibrated Zero\" \nglobal Variable"
      # "Bound to \"DeGaussing Finished\""
      # "Ensure that the correct value is displayed\n(2.49±0.05 (V))"
      n116 = shared-variable "NI-GenericDesktopPC-3A84958E\\Kopco PS Project Target Variables Library.lvlib\\DeGuassing Finished"(TRUE ("DeGuassing Finished")) -> ()  [unwired: 1 in, 1 out]
    }
    frame #6 {
      # "Bound to \"Needle Selection Finished\" \nshared global variable."
      # "Step 1 Selecting Needle & Sensor\n& PID Parameters"
      n117 = while {
        tunnel: ["Proceed with Selection"] -> w246
        tunnel: ["2. Needle:"] -> w245
        tunnel: ["1. Sensor:"] -> w244
        tunnel: ["3. PID Parameters:"] -> w243
        tunnel: ["4. Aggressiveness:"] -> w242
        stop <- "Proceed with Selection" stop-if-true
        # "Added on 1/16/2018"
      }
      n118 = shared-variable "NI-GenericDesktopPC-3A84958E\\Kopco PS Project Target Variables Library.lvlib\\Needle Selection Finished"(w246) -> ()  [unwired: 1 in, 1 out]
    }
    frame #7 {
      # "Step 1 Selecting Needle & Sensor\n& PID Parameters"
      # "1/5/2018\nGot rid of \"normal\" PID Gains, Only kept Aggressive..\n\nFrom now on, that name will be dropped."
      # "Needle Used no needed so far\nbut might be used in future versinos\n12/20/2017"
      # "More precisely measured Magnetic Sensor value for Sensors 1 & 2 on 11/28/2017"
      # "Older Magnetic Sensitivity Measured before 11/2017 for Sensor 2 very crudely\n0.003112 V/GS.\nPreviously sensor 2 zero was 2.4942892 V based on 10-minute experiments on 7/12/2017"
      # "Coupled with Shared Variable Sensor 1"
      # "Old parameters for HyMu80 were:\n0.095, 1E-5, 0 before 12/5/2017"
      n119 = case shown="1" w255 {
        tunnel: [T5 {"proportional gain (Kc)"=0.051, "integral time (Ti, min)"=3e-06, "derivative time (Td, min)"=0.0} ("PID gains HyMu80 #1 (Aggressive)") T5 {"proportional gain (Kc)"=0.051, "integral time (Ti, min)"=3.5e-06, "derivative time (Td, min)"=0.0} ("PID gains HyMu80 #2 (Aggressive)")] -> w257
        tunnel: [i8 1 ("Needle Used") i8 2 ("Needle Used")] -> w258
        frame 0, Default {
          # "HyMu80#1 (Aggressive) Parameters\nModified from 0.08 to 0.075 on 4/2/2018"
          # "D"
          # "I"
          # "P"
        }
        frame 1 {
          # "HyMu80#2 (Aggressive) Parameters\n12/21/2017\n\n\"HyMu80#2 PID Check Aggressive -40Gs Zero 100Gs 2.txt\"\nResponse Time ~ 21 ms"
          # "D"
          # "I"
          # "P"
        }
      }
      n120 = case shown="1" w254 {
        tunnel: [0.0029794 0.0030418] -> w256
        frame 0, Default {
          (unwired) 2.4837669
          # "Zero = 2.4837669 V"
          # "Sensor #1"
          # "Sensitivity = 2.9794 mV/GS"
        }
        frame 1 {
          (unwired) 2.4928421
          # "Zero = 2.4928421 V"
          # "Sensor #2"
          # "Sensor 2 = 3.0418 mV/GS"
        }
      }
      n121 = shared-variable "NI-GenericDesktopPC-3A84958E\\Kopco PS Project Target Variables Library.lvlib\\Sensor Sensitivity Core"(w256) -> ()  [unwired: 1 in, 1 out]
      n122 = shared-variable "NI-GenericDesktopPC-3A84958E\\Kopco PS Project Target Variables Library.lvlib\\Needle Used"(w258) -> ()  [unwired: 1 in, 1 out]
    }
    frame #8 {
      w269 = "1. SET-UP & RUN \"LIVE-FAST\" image acquisition in Nikon Elements. \n2. POSITION the magnetic needle in the glycerol sample within 100 micron of several beads. (Please refer to latest calibration protocol for more details). \n3. Click OK then follow the Steps 3:\n      1. CLICK \"Start Null Flux Adjustment.\"\n      2. Adjust the Magnetic Flux until beads are no longer attacted to the needle.\n      3. Select if you want the flux to stay running until the control sequence is used in Step 4\n      3. CLICK \"FINISH Null Flux Adjustment?\" to Move to Step 4 \n"  # 1. SET-UP & RUN "LIVE-FAST" image acquisition in Nikon Elements.  2. POSITION the magnetic needle in the glycerol sample within 100 micron of several beads. (Please refer to latest calibration protocol for more details).  3. Click OK then follow the Steps 3:       1. CLICK "Start Null Flux Adjustment."       2. Adjust the Magnetic Flux until beads are no longer attacted to the needle.       3. Select if you want the flux to stay running until the control sequence is used in Step 4       3. CLICK "FINISH Null Flux Adjustment?" to Move to Step 4
      n123 = One Button Dialog(message=w269, button name ("OK")="OK!") -> ()  [unwired: 1 out]
    }
    frame #9 {
      # "Bound to \"Flux RT Control\" \nglobal shared variable?"
      # "Step 2 Finding Null Flux in Real Time"
      n124 = while {
        tunnel: ["Start Null Flux Adjustment"] -> w274
        tunnel: [w275] -> w272
        tunnel: w273 -> [w275]
        stop <- "Start Null Flux Adjustment" stop-if-true
      }
      n125 = shared-variable "NI-GenericDesktopPC-3A84958E\\Kopco PS Project Target Variables Library.lvlib\\Flux RT Control"(w274) -> ()  [unwired: 1 in, 1 out]
    }
    frame #10 {
      w291 = -1 items=["default"=-1, "RSE"=10083, "NRSE"=10078, "Differential"=10106, "Pseudodifferential"=12529] ("Terminal Configuration")
      w296 = 12522 items=["Finite Samples"=10178, "Continuous Samples"=10123, "Hardware Timed Single Point"=12522]  # Sample Mode
      w302 = 10106 items=["default"=-1, "RSE"=10083, "NRSE"=10078, "Differential"=10106, "Pseudodifferential"=12529] ("Terminal Configuration")
      w305 = 12522 items=["Finite Samples"=10178, "Continuous Samples"=10123, "Hardware Timed Single Point"=12522]  # Sample Mode
      # "Step 2 Finding Null Flux in Real Time"
      # "Hardware-Time control loop cannot keep up\nwith 50,000 Hz frequence."
      # "Power Supply Control"
      # "Magnetic Flux Sensor Signals\nRelayed over three channels."
      n126 = shared-variable "NI-GenericDesktopPC-3A84958E\\Kopco PS Project Target Variables Library.lvlib\\Channels AI List"() -> (w277:string)  [unwired: 1 in, 1 out]
      n127 = shared-variable "NI-GenericDesktopPC-3A84958E\\Kopco PS Project Target Variables Library.lvlib\\Sampling Rate"() -> (w278:dbl)  [unwired: 1 in, 1 out]
      n128 = call-poly <vilib>:"DAQmx Create Virtual Channel.vi"("maximum value"=5.0 ("Max Voltage"), "minimum value"=0.0 ("Min Voltage"), "input terminal configuration"=w302, "physical channels"=w277) -> ("task out"=w303:refnum<k21>, "error out"=w304:errorcluster)  [unwired: 10 in]
      n129 = call-poly <vilib>:"DAQmx Create Virtual Channel.vi"("maximum value"=10.0, "minimum value"=-10.0, "output terminal configuration"=w291, "physical channels"="Dev2/ao0") -> ("task out"=w299:refnum<k21>, "error out"=w298:errorcluster)  [unwired: 10 in]
      n130 = call-poly <vilib>:"DAQmx Timing.vi"("task/channels in"=w303, "sample mode"=w305, "rate"=w278, "error in"=w304) -> ("task out"=w294:refnum<k21>, "error out"=w290:errorcluster)  [unwired: 10 in]
      n131 = call "Get Terminal Name with Device Prefix.vi"("error in"=w290, "Local Terminal Name"="ai/SampleClock", "task/channels in"=w294) -> ("error out"=w287:errorcluster, "Terminal Name with Device Prefix"=w289:tag, "task out"=w284:refnum<k21>)  [unwired: 6 in]
      n132 = call-poly <vilib>:"DAQmx Timing.vi"("task/channels in"=w299, "sample mode"=w296, "rate"=w278, "source"=w289, "error in"=w298) -> ("task out"=w286:refnum<k21>, "error out"=w285:errorcluster)  [unwired: 9 in]
      n133 = call <vilib>:"DAQmx Start Task.vi"("task/channels in"=w286, "error in"=w285) -> ("task out"=w282:refnum<k21>, "error out"=w295:errorcluster)  [unwired: 12 in]
      n134 = Merge Errors(w287, w295) -> (w283:errorcluster)
    }
    frame #11 {
      w318 = 30  # # of samples pushed to PID loop
      # "Bound to \"Null Flux Running Middle\" \nshared global variable."
      # "Bound to \"Null Flux Selected\"\nshared global variable"
      # "Step 2 Finding Null Flux in Real Time"
      # "Step 2 Finding Null Flux in Real Time"
      # "12/13/2017. Cannot turn on flux control sequence inside Real-time loop. That is why I have used the trigger in the Datalogger to turn th is on. \nOtherwise, it will remain off"
      # "PID is 30 times slower"
      n135 = shared-variable "NI-GenericDesktopPC-3A84958E\\Kopco PS Project Target Variables Library.lvlib\\Zero Flux Calibrated Core"() -> (w313:dbl)  [unwired: 1 in, 1 out]
      n136 = shared-variable "NI-GenericDesktopPC-3A84958E\\Kopco PS Project Target Variables Library.lvlib\\Sensor Sensitivity Core"() -> (w311:dbl)  [unwired: 1 in, 1 out]
      n137 = call-poly <vilib>:"DAQmx Create Timing Source.vi"("task/channels in"=w326, "sleep time (us)"=1.0, "error in"=w325) -> ("task out"=w332:refnum<k21>, "timing source out"=w329:string, "error out"=w330:errorcluster)  [unwired: 10 in]
      n138 = shared-variable "NI-GenericDesktopPC-3A84958E\\Kopco PS Project Target Variables Library.lvlib\\Sensor Index Flux Core"() -> (w306:i8)  [unwired: 1 in, 1 out]
      n139 = Reciprocal(x=w309) -> (1/x=w320:dbl)
      n140 = Multiply(x=w318, y=w320) -> (x*y=w319:dbl)
      n141 = node-c288(w329, w330) -> (w336:T2)  [unwired: 8 in]
      n142 = Initialize Array "Initialize Array"(0, 0 ("level 3 duration 0.1ms")) -> (w327:i32[])
      n143 = timed-loop {
        tunnel: w332 -> [w367]
        tunnel: [w362] -> w323
        tunnel: w324 -> [w366]
        tunnel: [w364] -> w322
        tunnel: w330 -> [w363]
        tunnel: [w353] -> w321
        timing: w336 -> [_]
        timing-out: [_] -> w335
        shift-right: [w349] -> _
        shift-left: 0 -> [w359]
        shift-right: [w356] -> _
        shift-left: w327 -> [w357]
        tunnel: w318 -> [w347]
        tunnel: w319 -> [w346]
        tunnel: w313 -> [w345]
        tunnel: w311 -> [w344]
        tunnel: [w339] -> w317
        tunnel: [w343] -> _
        tunnel: [w343] -> w316
        tunnel: [w342] -> w315
        tunnel: w312 -> [w341]
        tunnel: [w340] -> w307
        tunnel: w306 -> [w337]
        stop <- w343 continue-if-true
        # "Observed Flux (V)"
        # "Keep this control inside the loop so that changed in \nreal time under live imaging"
        # "Flux Sensor Calibrated Zero value (V)"
        n144 = node-c288() -> ()  [unwired: 1 in, 1 out]
        n145 = call-poly <vilib>:"DAQmx Read.vi"("task/channels in"=w367, "error in"=w363) -> ("task out"=w362:refnum<k21>, "data"=w354:dbl[], "error out"=w365:errorcluster)  [unwired: 11 in]
        n146 = Delete From Array "Choose 1st Channel"(array=w354, index=w337) -> (deleted portion=w358:dbl)  [unwired: 1 in, 1 out]
        n147 = Build Array (concatenate) "AI Array"(w358, w357) -> (w355:dbl[])
        n148 = Array Size(array=w355) -> (size(s)=w361:i32)
        n149 = Equal?(x=w361, y=w347) -> (x = y?=w360:bool)
        n150 = case shown="True" "2. Force Clamp?" {
          tunnel: [12.0921 ("x") -195.0 ("x")] -> w339
          frame False {
            # "Corrected Null\nFlux (Gs)"
          }
          frame True {
            (unwired) -172.0 ("x")
            # "-175Gs relative \nto null flux!\nInitial null flux = 3 Gs"
          }
        }
        n151 = Multiply(x=w339, y=w344) -> (x*y=w348:dbl)
        n152 = Add "Zero Offset"(x=w345, y=w348) -> (x+y=w352:dbl)
        n153 = case shown="True" w360 {
          tunnel: w346 -> [_ w382]
          tunnel: w352 -> [_ w387]
          tunnel: [w380 w385] -> w349
          tunnel: w359 -> [w380 _]
          tunnel: w355 -> [w379 w384]
          tunnel: [w379 w383] -> w356
          tunnel: w341 -> [_ w381]
          frame False {
          }
          frame True {
            # "Max/Min controller outputs"
            n154 = call-poly <vilib>:"Mean.vi"("X"=w384) -> ("mean"=w386:dbl)  [unwired: 1 out]
            n155 = call-poly <vilib>:"PID.vi"("reinitialize? (F)"=FALSE, "output range"=cluster{"output high":dbl, "output low":dbl} {"output high"=10.0, "output low"=-10.0}, "dt (s)"=w382, "PID gains"=w381, "process variable"=w386, "setpoint"=w387) -> ("output"=w385:dbl)  [unwired: 4 in, 1 out]
            n156 = Initialize Array(0, 0) -> (w383:i32[])
          }
        }
        n157 = case shown="True" "4. Stop Program" {
          tunnel: [w371 TRUE ("y")] -> w350
          tunnel: [w372 w374] -> w340
          tunnel: w349 -> [w372 w375]
          tunnel: [w371 "3. Keep Null Flux Running \n       Until Next Step?"] -> w342
          frame False {
            w371 = FALSE ("y")
          }
          frame True {
            # "A Toggle fixed the problem!"
            n158 = case shown="True" "3. Keep Null Flux Running \n       Until Next Step?" {
              tunnel: [0.0 ("output") w378] -> w374
              tunnel: w375 -> [_ w378]
              frame False {
                # "Reset AO at the end"
              }
              frame True {
                # "Keep Flux the same"
              }
            }
          }
        }
        n159 = call-poly <vilib>:"DAQmx Write.vi"("task/channels in"=w366, "data"=w340, "error in"=w365) -> ("task out"=w364:refnum<k21>, "error out"=w353:errorcluster)  [unwired: 10 in, 1 out]
        n160 = Unbundle By Name(w353) -> ("status"=w368:bool)  [unwired: 2 out]
        n161 = Not Or(1:w350, 2:w368) -> (0:w343:bool)
        n162 = node-c288() -> ()  [unwired: 1 in, 1 out]
      }
      n163 = node-c288(w335) -> ()  [unwired: 1 out]
      n164 = Not(x=w316) -> (.not. x?=w314:bool)
      n165 = shared-variable "NI-GenericDesktopPC-3A84958E\\Kopco PS Project Target Variables Library.lvlib\\Null Flux Running Middle"(w315) -> ()  [unwired: 1 in, 1 out]
      n166 = shared-variable "NI-GenericDesktopPC-3A84958E\\Kopco PS Project Target Variables Library.lvlib\\Zero Flux Observed GS"(w317) -> ()  [unwired: 1 in, 1 out]
      n167 = shared-variable "NI-GenericDesktopPC-3A84958E\\Kopco PS Project Target Variables Library.lvlib\\Null Flux Selected"(w314) -> ()  [unwired: 1 in, 1 out]
      n168 = shared-variable "NI-GenericDesktopPC-3A84958E\\Kopco PS Project Target Variables Library.lvlib\\Flux RT Control"(w316) -> ()  [unwired: 1 in, 1 out]
    }
    frame #12 {
      # "Zeroing the PS Output at the end with a STOP botton.\nReplacing it with a Toggle seemed to do the trick.\n \nSwitch the toggle \"mechanical action\" to \n\"Latch when Released\" so that it will reset to FALSE \nat the end every time."
      n169 = call <vilib>:"DAQmx Stop Task.vi"("task/channels in"=w401, "error in"=w399) -> ("task out"=w406:refnum<k21>, "error out"=w405:errorcluster)  [unwired: 12 in]
      n170 = call <vilib>:"DAQmx Clear Task.vi"("task in"=w406, "error in"=w405) -> ("error out"=w402:errorcluster)  [unwired: 13 in]
      n171 = Stop() -> ()  [unwired: 1 in]
      n172 = call <vilib>:"DAQmx Stop Task.vi"("task/channels in"=w400, "error in"=w402) -> ("task out"=w404:refnum<k21>, "error out"=w403:errorcluster)  [unwired: 12 in]
      n173 = call <vilib>:"DAQmx Clear Task.vi"("task in"=w404, "error in"=w403) -> ()  [unwired: 13 in, 1 out]
    }
  }
